vi "splitLinesIntoVolumes.vi"(10 "don't save lines for future":bool, 11 "Array of lines":T1[](array[typedef])) -> (2 "split lines":T2(array[cluster]), 3 "lines for future volume":T1[](array[typedef]))   [LabVIEW 2010]
uses:
  line_info.ctl
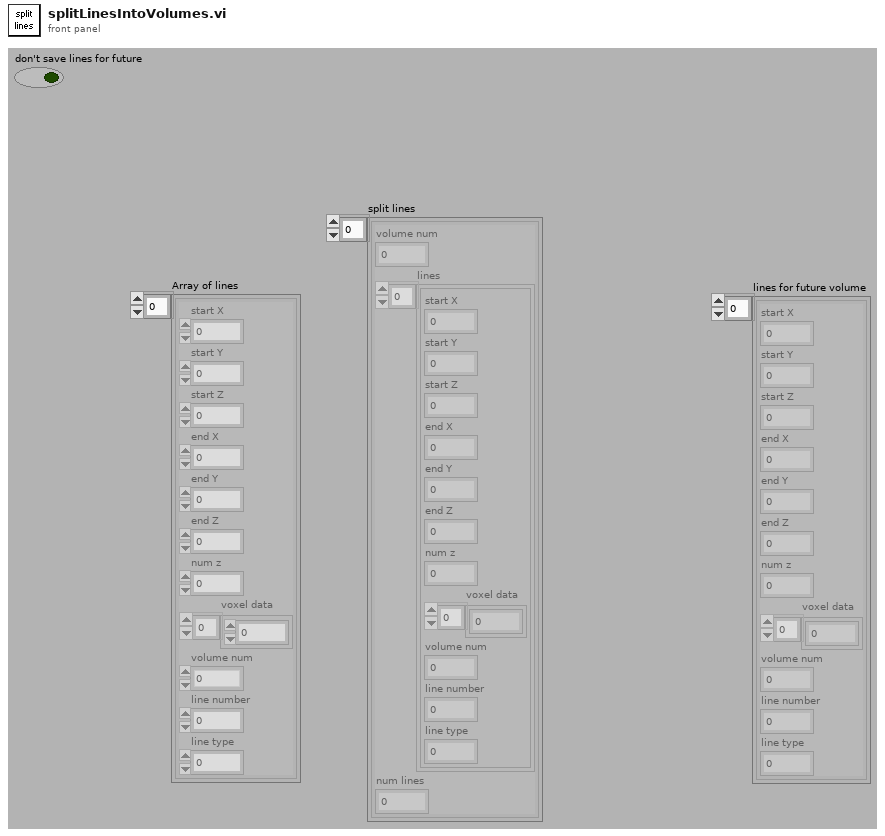
[diagram p1: front panel]
types:
  T1 = typedef "line_info.ctl" = cluster{"start X":i16, "start Y":i16, "start Z":i16, "end X":i16, "end Y":i16, "end Z":i16, "num z":u8, "voxel data":u32[], "volume num":u32, "line number":u16, "line type":u16}
  T2 = cluster{"volume num":u32, "lines":T1[], "num lines":u32}[]
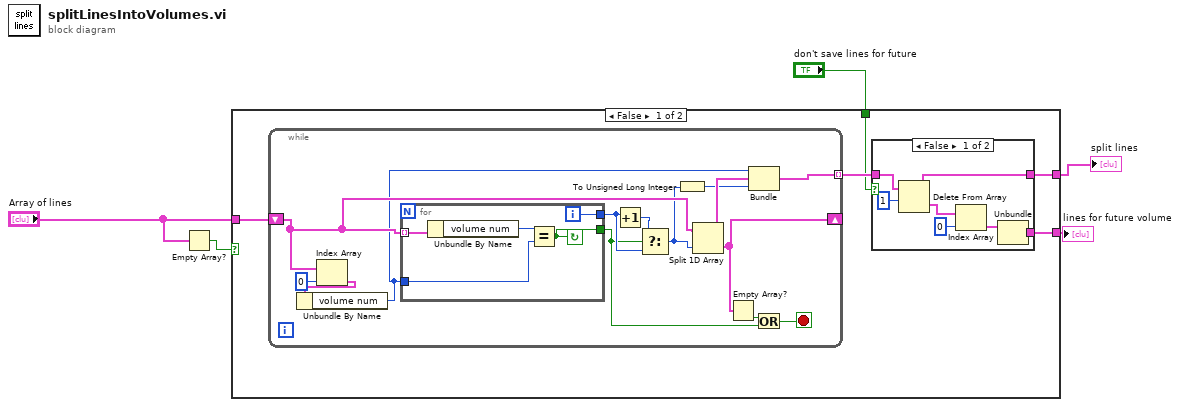
[diagram p0: block diagram]
diagram:
  n1 = Empty Array?(array="Array of lines") -> (empty?=w3:bool)
  n2 = case shown="False" w3 {
    tunnel: "Array of lines" -> [w10 w38]
    tunnel: [w8 _] -> w5
    tunnel: [w7 w38] -> w2
    tunnel: "don't save lines for future" -> [w6 _]
    frame False {
      n3 = while {
        shift-right: [w27] -> _
        shift-left: w10 -> [w28]
        tunnel: [w21] -> w9 mode=indexing
        stop <- w24 stop-if-true
        n4 = Index Array(array=w28, index=0) -> (element=w31:T1)
        n5 = Unbundle By Name(w31) -> ("volume num"=w23:u32)
        n6 = for {
          tunnel: w28 -> [w37] mode=indexing
          tunnel: w23 -> [w33]
          tunnel: [w36] -> w29
          tunnel: [w35] -> w25
          i -> [w36]
          stop <- w35 continue-if-true
          n7 = Unbundle By Name(w37) -> ("volume num"=w34:u32)
          n8 = Equal?(x=w34, y=w33) -> (x = y?=w35:bool)
        }
        n9 = Increment(x=w29) -> (x+1=w30:i32)
        n10 = Select(t=w30, s=w25, f=w29) -> (s? t:f=w20:i32)
        n11 = To Unsigned Long Integer(number=w20) -> (unsigned 32bit integer=w19:u32)
        n12 = Split 1D Array(array=w28, index=w20) -> (first subarray=w22:T1[], second subarray=w27:T1[])
        n13 = Empty Array?(array=w27) -> (empty?=w26:bool)
        n14 = Bundle("volume num"=w23, w22, w19) -> (w21:cluster{"volume num":u32, T1[], u32})  [unwired: 1 in]
        n15 = Or(x=w26, y=w25) -> (x .or. y?=w24:bool)
      }
      n16 = case shown="False" w6 {
        tunnel: w9 -> [w17 w18]
        tunnel: [w15 w18] -> w8
        tunnel: [w11 _] -> w7
        frame False {
          n17 = Delete From Array(array=w17, length=1) -> (deleted portion=w14:cluster{"volume num":u32, T1[], u32}[], array with subset deleted=w15:cluster{"volume num":u32, T1[], u32}[])  [unwired: 1 in]
          n18 = Index Array(array=w14, index=0) -> (element=w12:cluster{"volume num":u32, T1[], u32})
          n19 = Unbundle(w12) -> (w11:T1[])  [unwired: 2 out]
        }
        frame True {
        }
      }
    }
    frame True {
    }
  }
  "lines for future volume" <- w2
  "split lines" <- w5
